vi "Main.vi"   [LabVIEW 2019, in "ModuleB.lvlib"]
uses:
  ModuleB.lvlib
  Communication/ABComm/Message1/Message1.lvclass
  Utilities/StringUtilities/StringUtilities.lvlib
  Utilities/FileUtilities/FileUtilities.lvlib
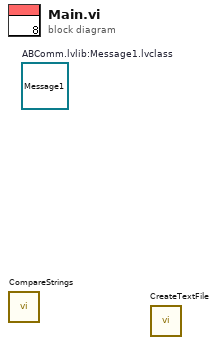
[diagram p0: block diagram]
diagram:
  (unwired) refnum<class "Message1.lvclass"> refnum  # ABComm.lvlib:Message1.lvclass
  n1 = call "CompareStrings.vi"() -> ()  [unwired: 12 in]
  n2 = call "CreateTextFile.vi"() -> ()  [unwired: 12 in]
